vi "Write Sim Image.vi"(8 "error in (no error)":errorcluster, 10 "Sim Image":path, 11 "Sim Camera Driver in":refnum<class "Sim Camera Driver.lvclass">) -> (0 "error out":errorcluster, 3 "Sim Camera Driver out":refnum<class "Sim Camera Driver.lvclass">)   [LabVIEW 2022 SP3, in "Sim Camera Driver.lvclass"]
uses:
  Sim Camera Driver.lvclass
  Sim Camera Driver.lvclass/Sim Camera Driver.ctl
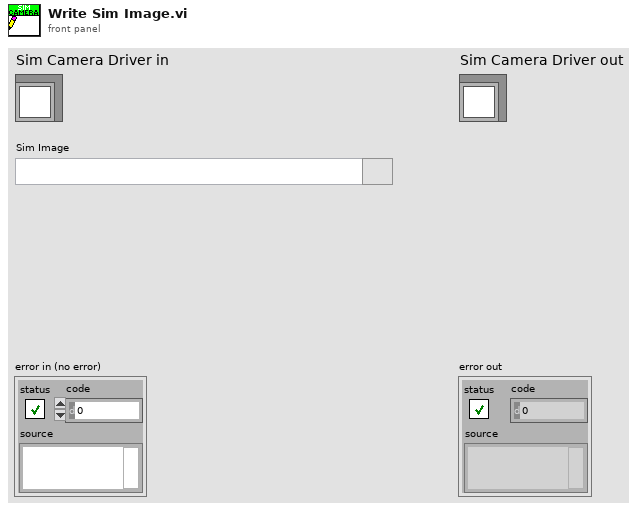
[diagram p1: front panel]
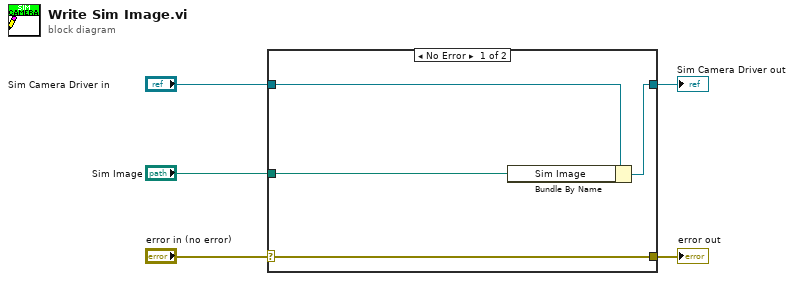
[diagram p0: block diagram]
diagram:
  n1 = case shown="No Error" "error in (no error)" {
    selector: "error in (no error)" -> [w9 w10]
    tunnel: [w9 w10] -> w4
    tunnel: [w7 w11] -> w2
    tunnel: "Sim Camera Driver in" -> [w8 w11]
    tunnel: "Sim Image" -> [w6 _]
    frame No Error {
      n2 = Bundle By Name(cluster=w8, "Sim Image"=w6) -> (w7:refnum<class "Sim Camera Driver.lvclass">)
    }
    frame Error {
    }
  }
  "error out" <- w4
  "Sim Camera Driver out" <- w2
